vi "Test.vi"   [LabVIEW 2020, in "E3610x.lvclass"]
uses:
  E3610x.lvclass
  C:/Sandbox/RF Bench/Source Code/WiSpry Test Framework/Instruments/Instrument.lvclass
  Instrument.lvclass/Instrument.ctl
  Instrument.lvclass
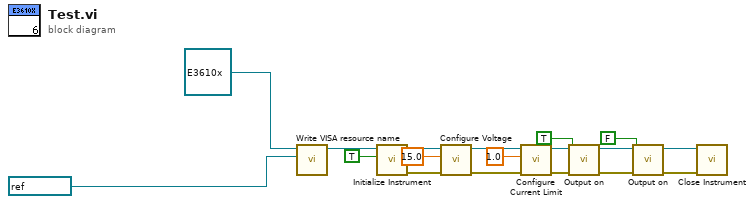
[diagram p0: block diagram]
diagram:
  n1 = call "Write VISA resource name.vi"("VISA resource name"=refnum<visa-resource-name> "DC20V", "Instrument in"=refnum<class "E3610x.lvclass"> refnum ("E3610x.lvclass")) -> ("Instrument out"=w16:refnum<class "E3610x.lvclass">)  [unwired: 9 in]
  n2 = call-dynamic "Initialize Instrument.vi"("Reset"=TRUE, "E3610x in"=w16) -> ("error out"=w14:errorcluster, "E3610x out"=w13:refnum<class "E3610x.lvclass">)  [unwired: 8 in]
  n3 = call-dynamic "Configure Voltage.vi"("error in (no error)"=w14, "Voltage"=15.0, "E3610x in"=w13) -> ("error out"=w11:errorcluster, "E3610x out"=w10:refnum<class "E3610x.lvclass">)  [unwired: 7 in]
  n4 = call-dynamic "Configure Current Limit.vi"("error in (no error)"=w11, "Current Limit"=1.0, "E3610x in"=w10) -> ("error out"=w8:errorcluster, "E3610x out"=w7:refnum<class "E3610x.lvclass">)  [unwired: 7 in]
  n5 = call-dynamic "Output on.vi"("error in (no error)"=w8, "Output On"=TRUE, "Power Supply in"=w7) -> ("error out"=w5:errorcluster, "Power Supply out"=w4:refnum<class "E3610x.lvclass">)  [unwired: 7 in]
  n6 = call-dynamic "Output on.vi"("error in (no error)"=w5, "Output On"=FALSE, "Power Supply in"=w4) -> ("error out"=w2:errorcluster, "Power Supply out"=w1:refnum<class "E3610x.lvclass">)  [unwired: 7 in]
  n7 = call-dynamic "Close Instrument.vi"("error in (no error)"=w2, "Instrument in"=w1) -> ()  [unwired: 8 in, 2 out]
